vi "matrici_v3.vi"() -> ()   [LabVIEW 2009]
panel:
  in  "stop":bool
  in  "Numar dde puncte":dbl(knob)=390.2948781423392 scale=0.0..500.0
  in  "Nr de perioade":dbl(knob)=1.4720771579664365 scale=0.0..25.0
  in  "Delta t":dbl(slide) scale=0.0..10.0
  out "Waveform Graph":cluster{"Slide":dbl, "Slide 2":dbl, dbl[]}(graph)={"Slide"=0.0, "Slide 2"=0.0, [0.0, 0.023714016745994635, 0.04741469593044595, 0.07108870749330436, 0.09472273637328865, 0.11830348999672478, 0.14181770575373695, 0.16525215845758598, 0.18859366778295963, 0.21182910567903146, 0.2349454037531186, 0.25792956062078587, 0.28076864921826217, 0.30344982407305654, 0.32596032852868423, 0.3482875019194402, 0.3704187866911833, 0.3923417354641282, 0.4140440180336705, 0.4355134283053091, 0.4567378911597648, 0.477705469244434, 0.49840436968735774, 0.5188229507299299, 0.5389497282746145, 0.5587733823439885, 0.578282763447479, 0.5974668988522109, 0.6163149987544427, 0.6348164623481147, 0.6529608837870996, 0.6707380580378002, 0.6881379866188049, 0.7051508832243695, 0.7217671792285653, 0.7379775290669969, 0.7537728154930615, 0.7691441547057964, 0.7840829013464273, 0.7985806533608087, 0.8126292567250232, 0.826220810031478, 0.8393476689329232, 0.8520024504418904, 0.8641780370831326, 0.8758675808967323, 0.8870645072896255, 0.897762518733373, 0.9079555983061032, 0.9176380130766315, 0.9268043173288536, 0.9354493556245999, 0.943568265703227, 0.9511564812163179, 0.9582097342959488, 0.9647240579550826, 0.9706957883187356, 0.9761215666846645, 0.9809983414124133, 0.9853233696396586, 0.9890942188248883, 0.9923087681155445, 0.9949652095408618, 0.997062049028732, 0.9985981072460199, 0.9995725202618604, 0.9999847400335617, 0.9998345347148435, 0.999121988786235, 0.99784750300756, 0.9960117941925363, 0.9936158948056157, 0.9906611523812908, 0.9871492287661965, 0.9830820991844313, 0.9784620511266253, 0.9732916830633774, 0.9675739029837891, 0.9613119267599126, 0.9545092763380367, 0.9471697777578253, 0.9392975590004239, 0.9308970476667437, 0.9219729684872306, 0.9125303406645169, 0.9025744750504529, 0.8921109711591051, 0.8811457140174013, 0.8696848708551923, 0.8577348876365954, 0.845302485434566, 0.8323946566507406, 0.8190186610826742, 0.8051820218406859, 0.790892521116609, 0.7761581958068225, 0.7609873329920321, 0.7453884652763348, 0.7293703659881975, 0.7129420442460387, 0.6961127398912, 0.6788919182911456, 0.6612892650158226, 0.6433146803901701, 0.6249782739258415, 0.6062903586352774, 0.5872614452313172, 0.5679022362156232, 0.5482236198592306, 0.5282366640786198, 0.5079526102107443, 0.48738286669052777, 0.4665390026343741, 0.445432741333306, 0.42407595365939404, 0.4024806513891754, 0.38065898044782914, 0.35862321407789605, 0.3363857459363968, 0.31395908312421866, 0.2913558391517038, 0.268588726844385, 0.24567055119286302, 0.22261420215085215, 0.19943264738543232, 0.17613892498360023, 0.15274613611920648, 0.12926743768441795, 0.10571603488983496, 0.0821051738374392, 0.058448134070538844, 0.03475822110490465, 0.01104875894530312, -0.012666917408376091, -0.03637546946116952, -0.06006356272506221, -0.08371787421874922, -0.10732509996093248, -0.13087196245292476, -0.15434521814636334, -0.17773166489182896, -0.201018149364176, -0.22419157446040908, -0.24723890666593126, -0.270147183385035, -0.29290352023149907, -0.3154951182752046, -0.33790927124068126, -0.3601333726535461, -0.3821549229308101, -0.40396153641106175, -0.4255409483205835, -0.44688102167147, -0.46796975408788233, -0.48879528455658494, -0.509345900097982, -0.529610042353889, -0.5495763140883434, -0.5692334855977955, -0.5885705010270691, -0.6075764845875495, -0.6262407466740904, -0.6445527898772108, -0.6625023148871884, -0.6800792262867417, -0.6972736382290293, -0.7140758799977849, -0.7304765014464539, -0.7464662783132728, -0.7620362174093063, -0.7771775616765174, -0.791881795113034, -0.8061406475628342, -0.8199460993671589, -0.8332903858750409, -0.8461660018104047, -0.8585657054932849, -0.8704825229127938, -0.881909751649538, -0.8928409646452857, -0.9032700138177591, -0.9131910335185252, -0.9225984438320322, -0.9314869537139433, -0.9398515639669961, -0.9476875700527221, -0.9549905647374358, -0.9617564405710115, -0.9679813921970523, -0.9736619184931499, -0.9787948245400345, -0.983377223418504, -0.9874065378331255, -0.9908805015617926, -0.9937971607303251, -0.9961548749113933, -0.9979523180471502, -0.999188479195051, -0.9998626630964403, -0.9999744905675904, -0.9995238987129657, -0.9985111409605981, -0.9969367869195505, -0.9948017220595488, -0.9921071472129644, -0.9888545778994264, -0.9850458434734406, -0.9806830860955001, -0.975768759527262, -0.9703056277514694, -0.9642967634173937, -0.9577455461126734, -0.950655660462521, -0.9430310940573648, -0.9348761352100942, -0.9261953705441676, -0.9169936824139422, -0.907276246158672, -0.8970485271917235, -0.8863162779266426, -0.8750855345418055, -0.8633626135854656, -0.851154108423116, -0.8384668855291596, -0.82530808062497, -0.8116850946655236, -0.7976055896768522, -0.7830774844466636, -0.7681089500705457, -0.7527084053562684, -0.7368845120887649, -0.7206461701584487, -0.7040025125556169, -0.6869629002337491, -0.6695369168445937, -0.6517343633479955, -0.6335652524995089, -0.6150398032188855, -0.596168434842612, -0.5769617612637207, -0.5574305849621807, -0.5375858909292214, -0.5174388404889994, -0.49700076502109664, -0.47628315958736966, -0.45529767646674274, -0.4340561186015692, -0.4125704329592615, -0.39085270381291704, -0.368915145944711, -0.3467700977758948, -0.3244300144272511, -0.30190746071391755, -0.2792151040785068, -0.2563657074665134, -0.233372122148002, -0.21024728048962363, -0.18700418868101212, -0.1636559194196676, -0.14021560455843388, -0.11669642771969703, -0.09311161688047566, -0.06947443693255945, -0.04579818222189092, -0.022096169071372268, 0.0016182717086794872, 0.02533180231823088, 0.04903108546915633, 0.07270279188658339, 0.09633360780572314, 0.11991024245997715, 0.14341943555611747, 0.16684796473231853, 0.19018265299486037, 0.21341037612931021, 0.2365180700820278, 0.2594927383078264, 0.2823214590796649, 0.30499139275626735, 0.32748978900356635, 0.3498039939659215, 0.3719214573830711, 0.3938297396488257, 0.41551651880751844, 0.4369695974842894, 0.45817690974529657, 0.4791265278840085, 0.49980666912974525, 0.5202057022747035, 0.5403121542157439, 0.5601147164072473, 0.5796022512214235, 0.5987637982124853, 0.617588580281176, 0.6360660097361717, 0.654185694248952, 0.6719374426988013, 0.6893112709046343, 0.7062974072404372, 0.7228862981311571, 0.7390686134259575, 0.7548352516458076, 0.7701773451024605, 0.7850862648859389, 0.7995536257177269, 0.8135712906669319, 0.8271313757267665, 0.840226254248783, 0.852848561232355, 0.8649911974670027, 0.8766473335252261, 0.8878104136036078, 0.8984741592100163, 0.9086325726948399, 0.9182799406242694, 0.9274108369937243, 0.9360201262796207, 0.9441029663277618, 0.9516548110767302, 0.9586714131147448, 0.9651488260685487, 0.9710834068229813, 0.9764718175699907, 0.981311027685928, 0.9855983154360726, 0.9893312695054274, 0.9925077903549234, 0.9951260914022717, 0.9971847000267966, 0.9986824583976879, 0.9996185241252036, 0.9999923707344583, 0.9998037879615305, 0.9990528818717216, 0.9977400747999019, 0.9958661051129751, 0.9934320267945956, 0.9904392088523726, 0.9868893345478942, 0.9827844004500048, 0.9781267153118676, 0.9729188987724421, 0.9671638798831147, 0.9608648954602973, 0.9540254882649363, 0.9466495050099433, 0.9387410941966722, 0.9303047037816661, 0.9213450786749746, 0.9118672580714553, 0.9018765726165641, 0.8913786414082193, 0.8803793688364294, 0.8688849412624703, 0.8569018235394613, 0.84443675537632, 0.8314967475471202, 0.8180890779479938, 0.8042212875038026, 0.7899011759268656, 0.7751367973301345, 0.7599364556972962, 0.7443087002123293, 0.728262320451152, 0.7118063414380762, 0.6949500185698209, 0.6777028324099736, 0.660074483356799, 0.6420748861874037, 0.62371416448134, 0.60500264492676, 0.585950851512334, 0.5665694996082131, 0.5468694899393409, 0.5268619024545133, 0.5065579900946514, 0.4859691724637644, 0.4651070294061751, 0.4439832944936359, 0.4226098484259609, 0.4009987123489312, 0.3791620410931929, 0.35711211633796625, 0.3348613397034254, 0.3124222257756047, 0.28980739506776926, 0.2670295669222232, 0.24410155235651815, 0.22103624685810072, 0.19784662313146786]}
  in  "t0":dbl(slide) scale=0.0..200.0
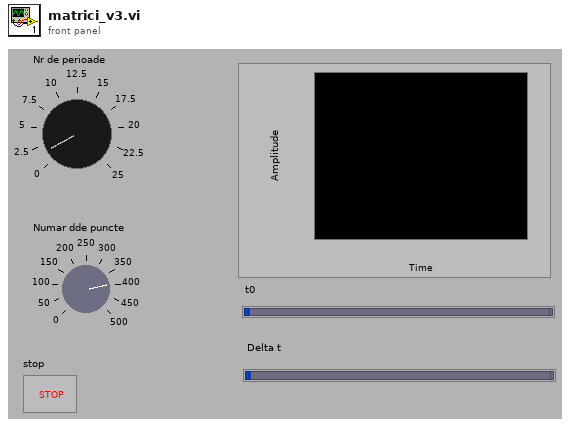
[diagram p1: front panel]
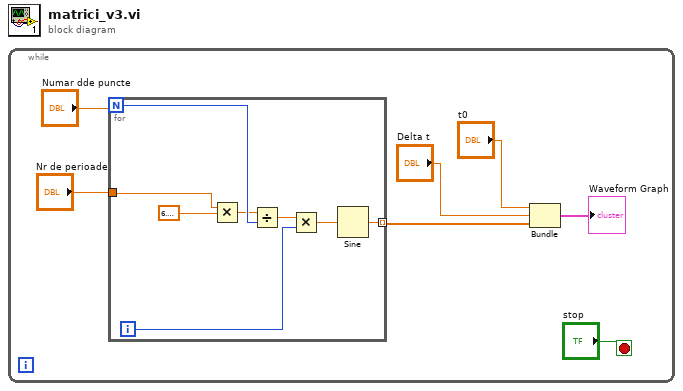
[diagram p0: block diagram]
diagram:
  n1 = while {
    stop <- "stop" stop-if-true
    n2 = for {
      N: "Numar dde puncte" -> [w14]
      tunnel: [w15] -> w3 mode=indexing
      tunnel: "Nr de perioade" -> [w9]
      i -> [w12]
      n3 = Multiply(x=w9, y=6.283185307179586) -> (x*y=w10:dbl)
      n4 = Divide(x=w10, y=w14) -> (x/y=w13:dbl)
      n5 = Multiply(x=w13, y=w12) -> (x*y=w11:dbl)
      n6 = Sine(x=w11) -> (sin(x)=w15:dbl)
    }
    n7 = Bundle("t0"="t0", "Delta t"="Delta t", w3) -> (→"Waveform Graph":cluster{"t0":dbl, "Delta t":dbl, dbl[]})  [unwired: 1 in]
  }
